vi "PC_UI.vi"() -> ()   [LabVIEW 2023]
doc: "Provides a basic example of a PC user interface that uses network streams to connect to a remote system.JKI Network Streams Connection 1.1.1.15\nJavier Ruiz - JKI\nCopyright (c) 2020, JKI\n\nThis library is provided \"AS IS\" ,WITHOUT WARRANTIES OR CONDITIONS OF ANY KIND, either express or implied."
uses:
  NetworkConnection.lvclass
  NetworkCommand.ctl
  PublicSettings.ctl
panel:
  in  "Stop":bool
  out "Incoming Messages":T1[](array[typedef])
  out "Timed Out?":bool
  in  "SEND":bool
  in  "Message To Send":T2={"Command"="Cmd From PC", "Arguments"=variant(string "Arguments are variants. Wire anything!"), " Msg Id"=0}
  in  "Settings":T3={"My Name"="PC", "Remote IP Address"="localhost", "Remote Name"="RT"}
  out "Connected?":bool
  # "JKI Network Stream 2-Way Communication Example\nPC Endpoint"
  # "Instructions: \n- Configure the settings below before running the VI: \n   IP Address is only needed on one end \n- Run the other endpoint.\n- If settings are the same the code will reconnect automatically\n- Type a Cmd Name and Click Send\n- Send from the other endpoint to see messages arrive here"
  # "*Arguments are variants\nso you can wire anything!"
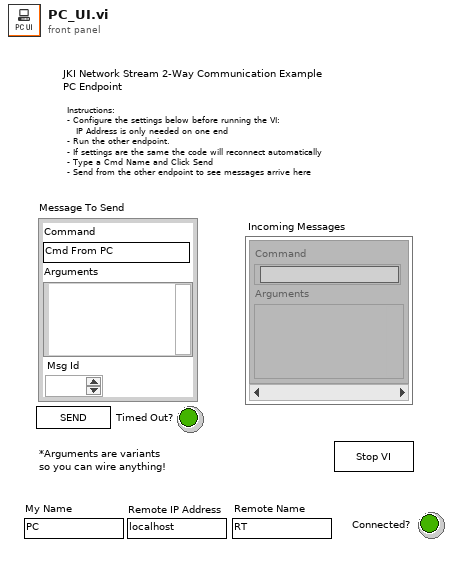
[diagram p1: front panel]
types:
  T1 = typedef "NetworkConnection.lvclass/NetworkCommand.ctl" = cluster{"Command":string, "Arguments":variant}
  T2 = typedef "NetworkConnection.lvclass/NetworkCommand--Cluster.ctl" = cluster{"Command":string, "Arguments":variant, " Msg Id":i32}
  T3 = typedef "NetworkConnection.lvclass/PublicSettings.ctl" = cluster{"My Name":string, "Remote IP Address":string, "Remote Name":string}
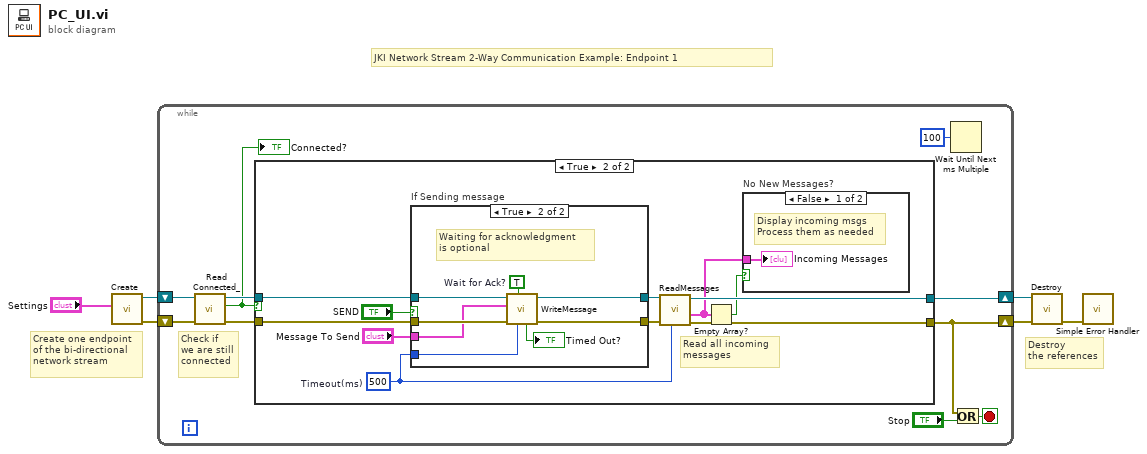
[diagram p0: block diagram]
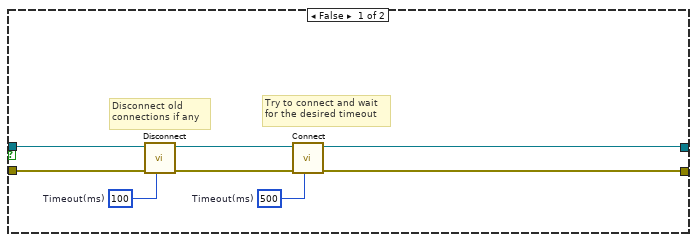
[diagram p2: hidden frame]
diagram:
  # "Destroy\nthe references"
  # "Create one endpoint\nof the bi-directional\nnetwork stream"
  # "JKI Network Stream 2-Way Communication Example: Endpoint 1"
  n1 = call "Create.vi"("Settings"="Settings") -> ("error out"=w3:errorcluster, "NetworkConnection out"=w5:refnum<class "NetworkConnection.lvclass">)  [unwired: 9 in]
  n2 = while {
    shift-right: [w12] -> w4
    shift-left: w5 -> [w16]
    shift-right: [w8] -> w2
    shift-left: w3 -> [w15]
    stop <- w7 stop-if-true
    # "Check if\nwe are still\nconnected"
    n3 = call "Read Connected_.vi"("error in (no error)"=w15, "NetworkConnection in"=w16) -> ("error out"=w14:errorcluster, "Connected?"=w10:bool, "NetworkConnection out"=w13:refnum<class "NetworkConnection.lvclass">)  [unwired: 7 in]
    "Connected?" <- w10
    n4 = case shown="True" w10 {
      tunnel: w14 -> [w19 w31]
      tunnel: w13 -> [w21 w32]
      tunnel: [w22 w35] -> w12
      tunnel: [w23 w34] -> w8
      frame False {
        w17 = 100  # Timeout(ms)
        w24 = 500  # Timeout(ms)
        # "Try to connect and wait\nfor the desired timeout"
        # "Disconnect old\nconnections if any"
        n5 = call "Disconnect.vi"("Timeout ms (1000)"=w17, "error in (no error)"=w19, "NetworkConnection in"=w21) -> ("error out"=w18:errorcluster, "NetworkConnection out"=w20:refnum<class "NetworkConnection.lvclass">)  [unwired: 7 in]
        n6 = call "Connect.vi"("Timeout(ms)"=w24, "error in (no error)"=w18, "NetworkConnection in"=w20) -> ("error out"=w23:errorcluster, "NetworkConnection out"=w22:refnum<class "NetworkConnection.lvclass">)  [unwired: 6 in, 1 out]
      }
      frame True {
        w29 = 500  # Timeout(ms)
        # "Read all incoming\nmessages"
        n7 = case "If Sending message" shown="True" "SEND" {
          tunnel: w32 -> [w38 w46]
          tunnel: w31 -> [w37 w45]
          tunnel: "Message To Send" -> [_ w44]
          tunnel: w29 -> [_ w43]
          tunnel: [w37 w40] -> w28
          tunnel: [w38 w39] -> w27
          frame False {
          }
          frame True {
            w42 = TRUE  # Wait for Ack?
            # "Waiting for acknowledgment\nis optional"
            n8 = call "WriteMessage.vi"("Timeout(ms)"=w43, "Wait for Ack? (false)"=w42, "error in (no error)"=w45, "Message"=w44, "NetworkConnection in"=w46) -> ("error out"=w40:errorcluster, "NetworkConnection out"=w39:refnum<class "NetworkConnection.lvclass">, "Timed Out?"=→"Timed Out?":bool)  [unwired: 3 in, 1 out]
          }
        }
        n9 = call "ReadMessages.vi"("Timeout(ms)"=w29, "error in (no error)"=w28, "NetworkConnection in"=w27) -> ("error out"=w34:errorcluster, "Messages"=w25:T1[], "NetworkConnection out"=w35:refnum<class "NetworkConnection.lvclass">)  [unwired: 4 in, 2 out]
        n10 = Empty Array?(array=w25) -> (empty?=w26:bool)
        n11 = case "No New Messages?" shown="False" w26 {
          tunnel: w25 -> [w36 _]
          frame False {
            # "Display incoming msgs\nProcess them as needed"
            "Incoming Messages" <- w36
          }
          frame True {
          }
        }
      }
    }
    n12 = Wait Until Next ms Multiple(millisecond multiple=u32 100) -> ()  [unwired: 1 out]
    n13 = Or(x=w8, y="Stop") -> (x .or. y?=w7:bool)
  }
  n14 = call "Destroy.vi"("error in (no error)"=w2, "NetworkConnection in"=w4) -> ("error out"=w1:errorcluster)  [unwired: 8 in, 1 out]
  n15 = call <vilib>:"Simple Error Handler.vi"("error in (no error)"=w1) -> ()  [unwired: 4 in, 5 out]
